vi "calc.vi"() -> ()   [LabVIEW 2022 SP3]
uses:
  ctl3.ctl
panel:
  in  ". 2":bool
  in  "backspace":bool
  in  "+/-":bool
  in  "stop":bool
  in  "String":string
  in  "0":bool
  in  "clr":bool
  in  "mul":bool
  in  "div":bool
  in  "add":bool
  in  "sub":bool
  in  "1":bool
  in  "8":bool
  in  "9":bool
  in  "6":bool
  in  "5":bool
  in  "7":bool
  in  "eql":bool
  in  "4":bool
  in  "2":bool
  in  "3":bool
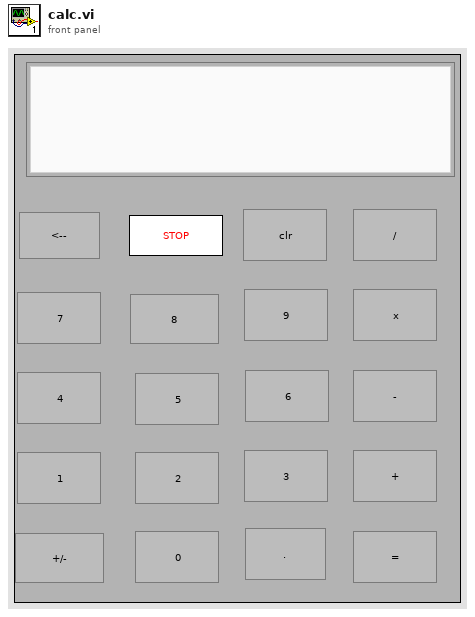
[diagram p1: front panel]
types:
  T1 = typedef "ctl3.ctl" = enum16{"Poll", "Intitalize", "Update Display", "Calculate", "Error", "Stop", "spliting", "Exit"}
  T2 = cluster{"a":string, "b":string, "Operand":string, "values":string, "String":refnum<vi>}
  T3 = typedef "eventvkey.ctl" = enum16{"ASCII", "Enter", "Return", "Shift", "Ctrl", "Alt", "Cmd", "Opt", "Caps", "NumLock", "Clear", "Break", "Up", "Down", "Left", "Right", "Insert", "Delete", "Home", "End", "PageUp", "PageDown", "Escape", "Help", "Pause", "ScrollLock", "F1", "F2", "F3", "F4", "F5", "F6", "F7", "F8", "F9", "F10", "F11", "F12", "F13", "F14", "F15", "F16", "F17", "F18", "F19", "F20", "F21", "F22", "F23", "F24", "Play", "VolumeUp", "VolumeDown", "Mute", "Two Byte Char"}
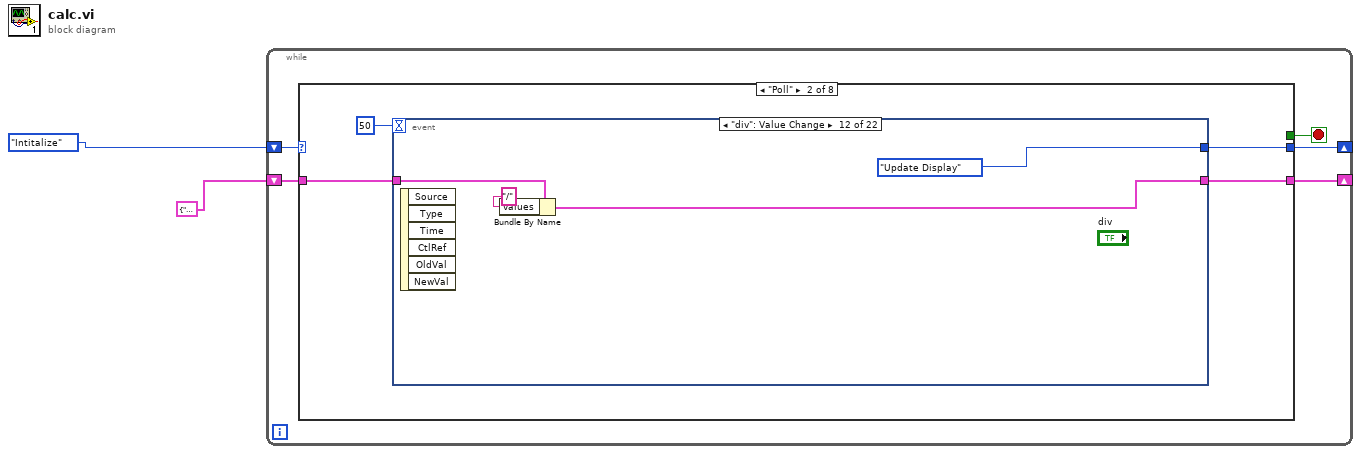
[diagram p0: block diagram]
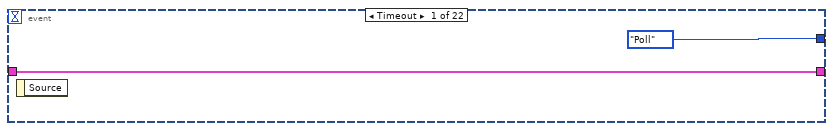
[diagram p3: hidden frame]
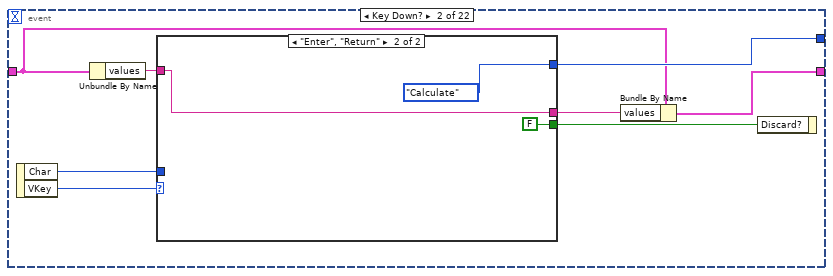
[diagram p4: hidden frame]
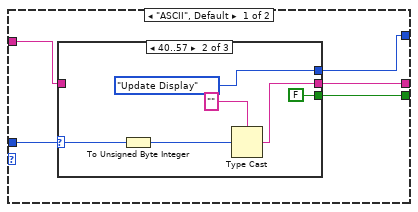
[diagram p5: hidden frame]
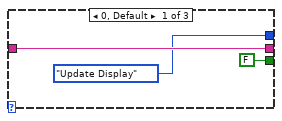
[diagram p6: hidden frame]
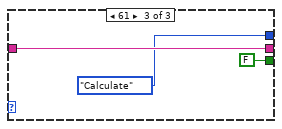
[diagram p7: hidden frame]
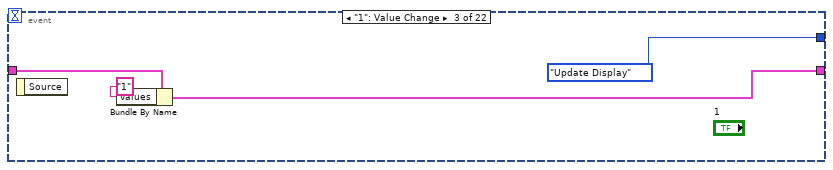
[diagram p8: hidden frame]
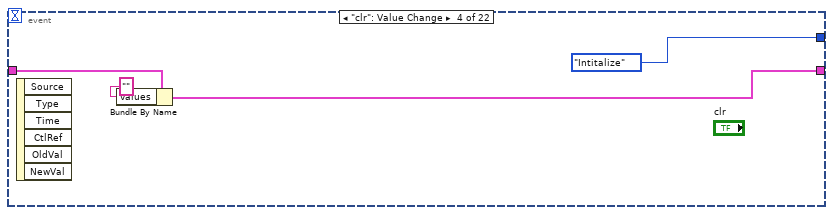
[diagram p9: hidden frame]
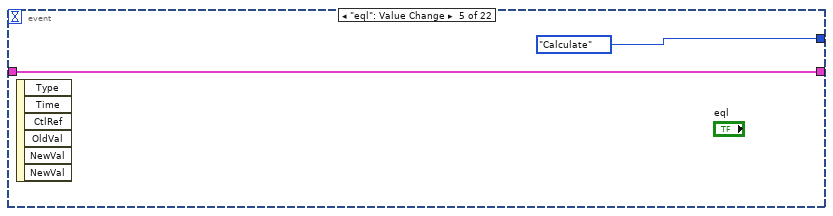
[diagram p10: hidden frame]
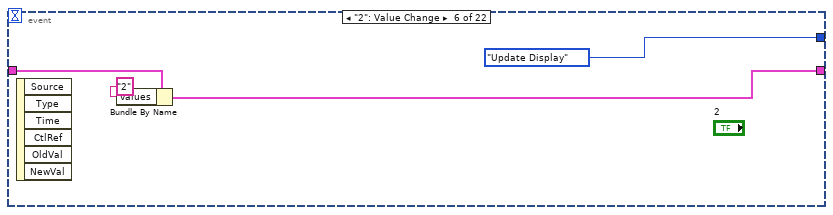
[diagram p11: hidden frame]
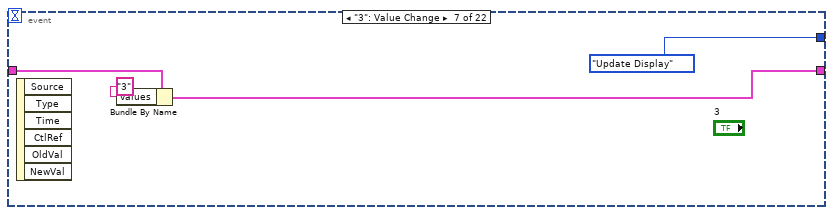
[diagram p12: hidden frame]
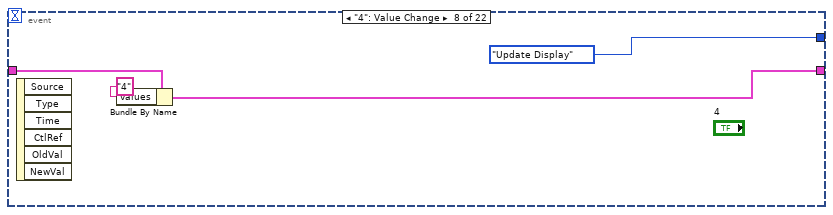
[diagram p13: hidden frame]
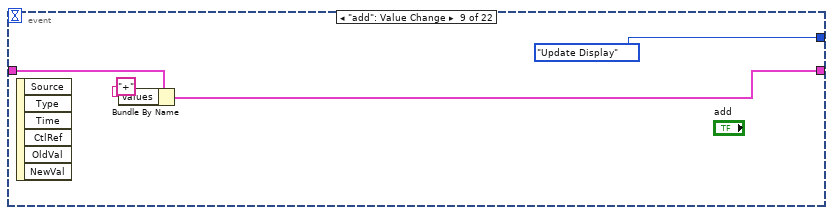
[diagram p14: hidden frame]
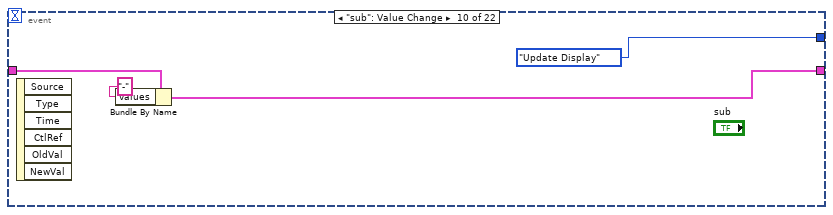
[diagram p15: hidden frame]
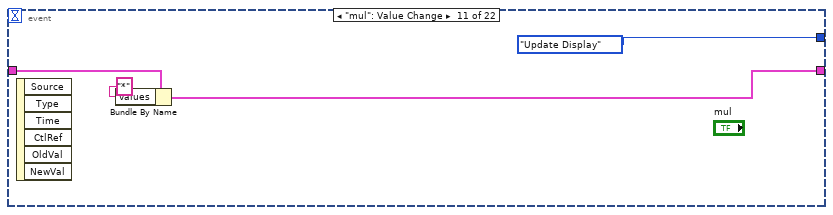
[diagram p16: hidden frame]
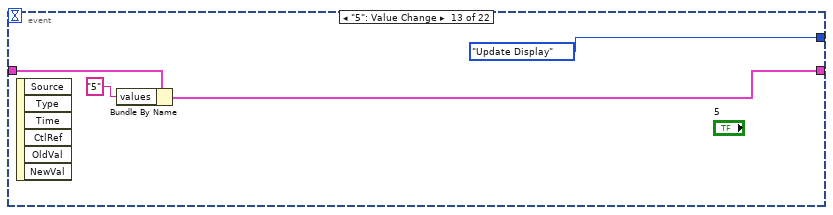
[diagram p17: hidden frame]
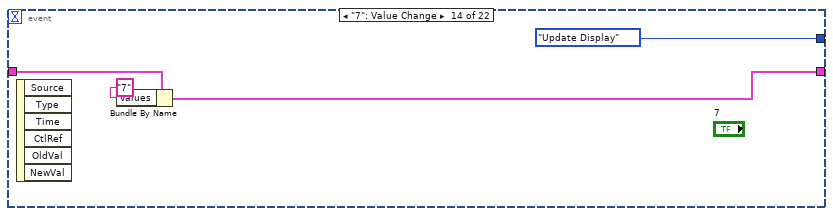
[diagram p18: hidden frame]
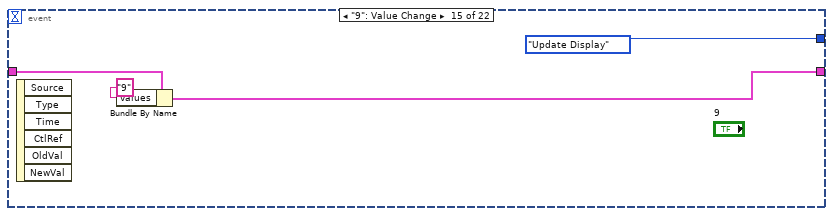
[diagram p19: hidden frame]
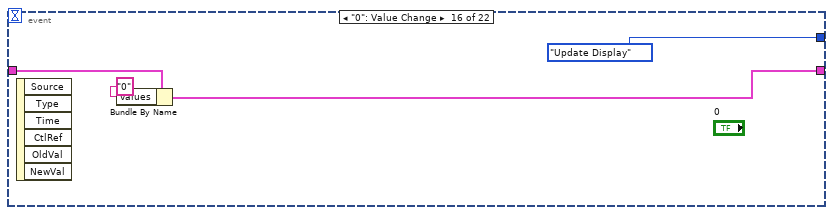
[diagram p20: hidden frame]
diagram:
  n1 = while {
    shift-right: [w3] -> _
    shift-left: T2 {"a"="", "b"="", "Operand"="", "values"="", "String"=refnum} -> [w7]
    shift-right: [w4] -> _
    shift-left: ctl3."Intitalize" -> [w5]
    stop <- w6 stop-if-true
    n2 = case shown="\"Poll\"" w5 {
      tunnel: [w8 w11 w124 w129 w137 w139 w144 w145] -> w3
      tunnel: w7 -> [w8 w12 w128 w129 w137 w139 w144 w145]
      tunnel: [_ _ _ _ _ _ _ TRUE ("stop")] -> w6
      tunnel: [_ w10 ctl3."Poll" _ ctl3."Poll" ctl3."Poll" ctl3."Poll" _] -> w4
      frame "Exit" {
      }
      frame "Poll" {
        n3 = event shown="[11] \"div\": Value Change" {
          selector: _ -> [_ _ _ _ _ _ _ _ _ _ _ _ _ _ _ _ _ _ _ _ _ _]
          dyn-events: _ -> [_ _ _ _ _ _ _ _ _ _ _ _ _ _ _ _ _ _ _ _ _ _]
          timeout: 50 -> [_ _ _ _ _ _ _ _ _ _ _ _ _ _ _ _ _ _ _ _ _ _]
          tunnel: w12 -> [w14 w17 w46 w50 w52 w56 w59 w63 w68 w72 w76 w80 w83 w87 w91 w95 w99 w103 w106 w110 w115 w119]
          tunnel: [w14 w15 w45 w49 w52 w54 w58 w62 w66 w70 w74 w78 w82 w86 w90 w94 w98 w102 w106 w110 w114 w117] -> w11
          tunnel: [ctl3."Poll" w20 ctl3."Update Display" ctl3."Intitalize" ctl3."Calculate" ctl3."Update Display" ctl3."Update Display" ctl3."Update Display" ctl3."Update Display" ctl3."Update Display" ctl3."Update Display" ctl3."Update Display" ctl3."Update Display" ctl3."Update Display" ctl3."Update Display" ctl3."Update Display" ctl3."Update Display" ctl3."Update Display" ctl3."Stop" ctl3."spliting" ctl3."Update Display" ctl3."Update Display"] -> w10
          event Timeout {
            n4 = event-data() -> ()  [unwired: 1 in, 1 out]
          }
          event Key Down? {
            n5 = event-data() -> ("Char"=w22:i16, "VKey"=w21:T3)  [unwired: 1 in]
            n6 = Unbundle By Name(w17) -> ("values"=w18:string)
            n7 = case shown="\"Enter\", \"Return\"" w21 {
              tunnel: w22 -> [w27 _]
              tunnel: w18 -> [w25 w42]
              tunnel: [w24 w42] -> w16
              tunnel: [w26 ctl3."Calculate"] -> w20
              tunnel: [w23 FALSE] -> w19
              frame "ASCII", Default {
                n8 = case shown="40..57" w27 {
                  selector: w27 -> [_ w33 _]
                  tunnel: [ctl3."Update Display" ctl3."Update Display" ctl3."Calculate"] -> w26
                  tunnel: w25 -> [w30 _ w39]
                  tunnel: [w30 w35 w39] -> w24
                  tunnel: [FALSE FALSE FALSE] -> w23
                  frame 0, Default {
                  }
                  frame 40..57 {
                    n9 = To Unsigned Byte Integer(number=w33) -> (unsigned 8bit integer=w32:u8)
                    n10 = Type Cast(type="", x=w32) -> (*(type *) &x=w35:string)
                  }
                  frame 61 {
                  }
                }
              }
              frame "Enter", "Return" {
              }
            }
            n11 = Bundle By Name(cluster=w17, "values"=w16) -> (w15:T2)
            n12 = event-data("Discard?"=w19) -> ()  [unwired: 1 in, 1 out]
          }
          event "1": Value Change {
            n13 = event-data() -> ()  [unwired: 1 in, 1 out]
            n14 = Bundle By Name(cluster=w46, "values"="1" ("a")) -> (w45:T2)
          }
          event "clr": Value Change {
            n15 = event-data() -> ()  [unwired: 1 in, 6 out]
            n16 = Bundle By Name(cluster=w50, "values"="" ("a")) -> (w49:T2)
          }
          event "eql": Value Change {
            n17 = event-data() -> ()  [unwired: 1 in, 6 out]
          }
          event "2": Value Change {
            n18 = event-data() -> ()  [unwired: 1 in, 6 out]
            n19 = Bundle By Name(cluster=w56, "values"="2" ("a")) -> (w54:T2)
          }
          event "3": Value Change {
            n20 = event-data() -> ()  [unwired: 1 in, 6 out]
            n21 = Bundle By Name(cluster=w59, "values"="3" ("a")) -> (w58:T2)
          }
          event "4": Value Change {
            n22 = event-data() -> ()  [unwired: 1 in, 6 out]
            n23 = Bundle By Name(cluster=w63, "values"="4" ("a")) -> (w62:T2)
          }
          event "add": Value Change {
            n24 = event-data() -> ()  [unwired: 1 in, 6 out]
            n25 = Bundle By Name(cluster=w68, "values"="+" ("Display")) -> (w66:T2)
          }
          event "sub": Value Change {
            n26 = event-data() -> ()  [unwired: 1 in, 6 out]
            n27 = Bundle By Name(cluster=w72, "values"="-" ("Display")) -> (w70:T2)
          }
          event "mul": Value Change {
            n28 = event-data() -> ()  [unwired: 1 in, 6 out]
            n29 = Bundle By Name(cluster=w76, "values"="*" ("Display")) -> (w74:T2)
          }
          event "div": Value Change {
            n30 = event-data() -> ()  [unwired: 1 in, 6 out]
            n31 = Bundle By Name(cluster=w80, "values"="/" ("Display")) -> (w78:T2)
          }
          event "5": Value Change {
            n32 = event-data() -> ()  [unwired: 1 in, 6 out]
            n33 = Bundle By Name(cluster=w83, "values"="5" ("a")) -> (w82:T2)
          }
          event "7": Value Change {
            n34 = event-data() -> ()  [unwired: 1 in, 6 out]
            n35 = Bundle By Name(cluster=w87, "values"="7" ("a")) -> (w86:T2)
          }
          event "9": Value Change {
            n36 = event-data() -> ()  [unwired: 1 in, 6 out]
            n37 = Bundle By Name(cluster=w91, "values"="9" ("a")) -> (w90:T2)
          }
          event "0": Value Change {
            n38 = event-data() -> ()  [unwired: 1 in, 6 out]
            n39 = Bundle By Name(cluster=w95, "values"="0" ("a")) -> (w94:T2)
          }
          event "8": Value Change {
            n40 = event-data() -> ()  [unwired: 1 in, 6 out]
            n41 = Bundle By Name(cluster=w99, "values"="8" ("a")) -> (w98:T2)
          }
          event "6": Value Change {
            n42 = event-data() -> ()  [unwired: 1 in, 6 out]
            n43 = Bundle By Name(cluster=w103, "values"="6" ("a")) -> (w102:T2)
          }
          event "stop": Value Change {
            n44 = event-data() -> ()  [unwired: 1 in, 6 out]
          }
          event "backspace": Value Change {
            n45 = event-data() -> ()  [unwired: 1 in, 1 out]
            n46 = Unbundle By Name(w110) -> ("String"=w109:refnum<vi>)
            n47 = property class="Str"(reference=w109) -> ("Value"=w111:string)  [unwired: 1 in, 2 out]
            n48 = call "backspace.vi"("string"=w111) -> ("result string"=w108:string)  [unwired: 10 in]
            n49 = property class="Str"(reference=w109, "Value"=w108) -> ()  [unwired: 1 in, 2 out]
          }
          event "+/-": Value Change {
            n50 = event-data() -> ()  [unwired: 1 in, 6 out]
            n51 = Bundle By Name(cluster=w115, "values"="+\\-" ("a")) -> (w114:T2)
          }
          event ". 2": Value Change {
            n52 = event-data() -> ()  [unwired: 1 in, 6 out]
            n53 = Bundle By Name(cluster=w119, "values"="." ("a")) -> (w117:T2)
          }
        }
      }
      frame "Intitalize", Default {
        n54 = control-ref of="String"() -> (w121:refnum<vi>)
        n55 = property on="String" class="Str"("Value"="" ("String")) -> ()  [unwired: 2 in, 2 out]
        n56 = Bundle By Name(cluster=w128, "a"="", "b"="", "Operand"="", "values"="" ("Display"), "String"=w121) -> (w124:T2)
      }
      frame "Error" {
      }
      frame "Calculate" {
        n57 = Match Pattern(string="String", regular expression="[ +-*/]") -> (before substring=w135:string, match substring=w133:string, after substring=w134:string)  [unwired: 1 in, 1 out]
        n58 = call "calucation.vi"("String 2"=w134, "String"=w133, "String 3"=w135) -> ("String 4"=w136:string)  [unwired: 8 in]
        n59 = property on="String" class="Str"("Value"=w136) -> ()  [unwired: 2 in, 2 out]
      }
      frame "Update Display" {
        n60 = Unbundle By Name(w139) -> ("values"=w141:string)
        n61 = property on="String" class="Str"() -> ("Value"=w142:string)  [unwired: 2 in, 2 out]
        n62 = Concatenate Strings(w142, w141) -> (w140:string)
        n63 = property on="String" class="Str"("Value"=w140) -> ()  [unwired: 2 in, 2 out]
      }
      frame "spliting" {
      }
      frame "Stop" {
      }
    }
  }
